vi "ATM main.vi"() -> ()   [LabVIEW 2017]
doc: "This VI is the main VI of the ATM simulator. This VI performs the all operation of the ATM machine as per the requirements."
panel:
  out "String":string
  out "Error Out":errorcluster
  in  "Mehr Buttons":cluster{"L1":bool, "L2":bool, "L3":bool}
  out "Display":string
  out "Menü 2":T1
  out "Menü 1":T1
  in  "Buttons":cluster{"L1":bool, "L2":bool, "L3":bool}
  in  "Enter":bool
  in  "Eingabe  Feld":string
  in  "Karteneingabe":bool
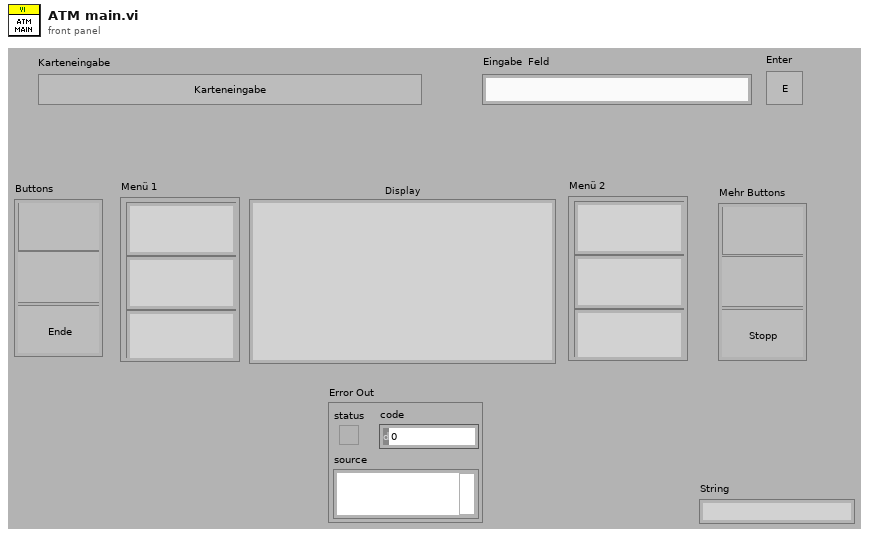
[diagram p1: front panel]
types:
  T1 = cluster{"LM1":string, "LM2":string, "LM3":string}
  T2 = enum8{"Enabled", "Disabled", "Disabled and Grayed Out"}
  T3 = cluster{"amount":string[], "accno":string[], "lst name":string[], "first name":string[]}
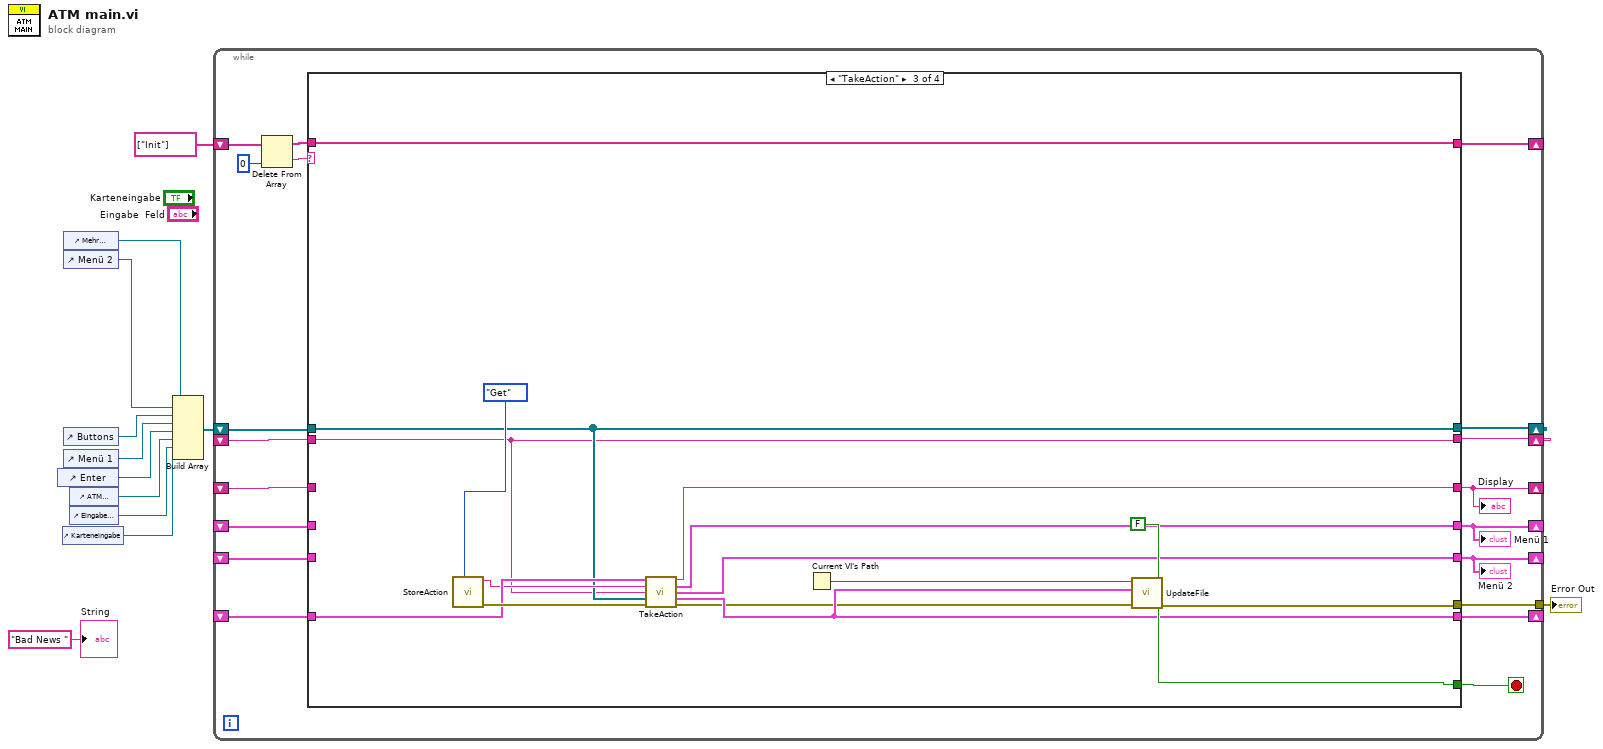
[diagram p0: block diagram]
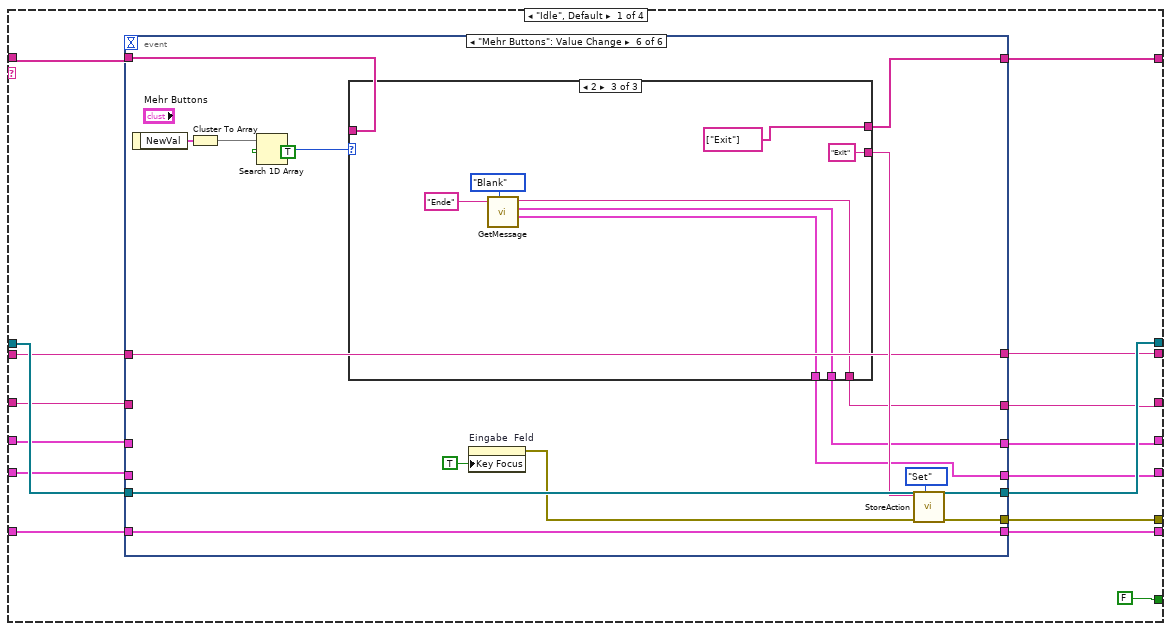
[diagram p2: hidden frame]
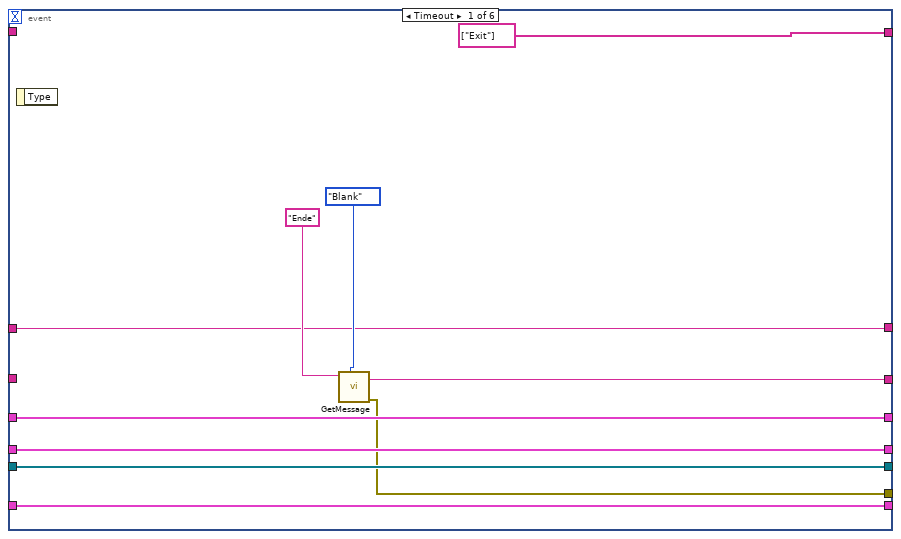
[diagram p3: hidden frame]
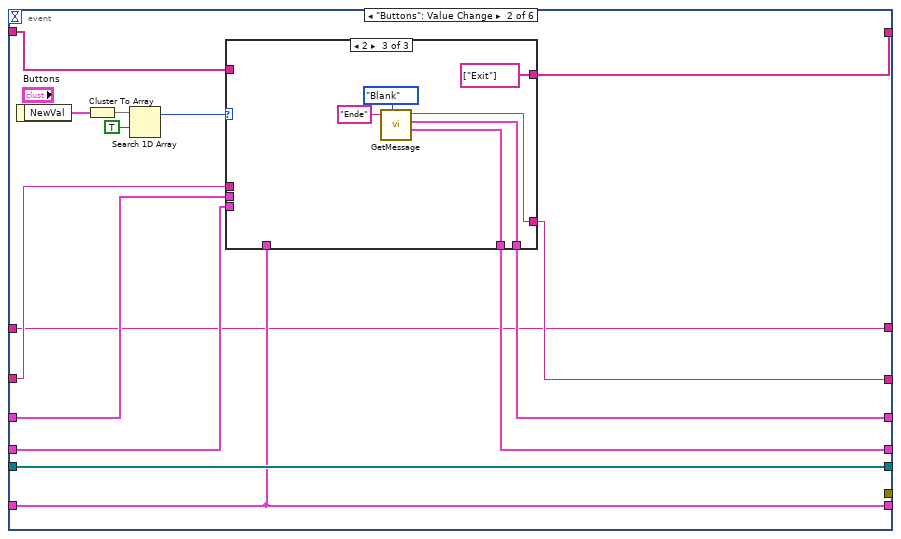
[diagram p4: hidden frame]
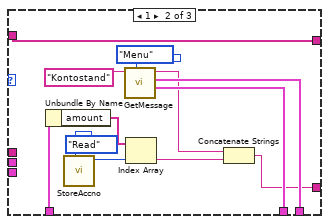
[diagram p6: hidden frame]
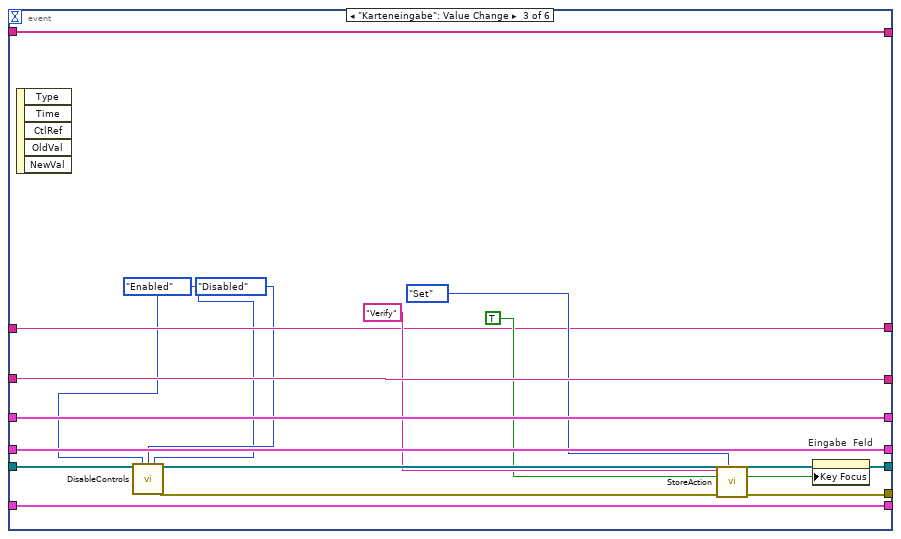
[diagram p7: hidden frame]
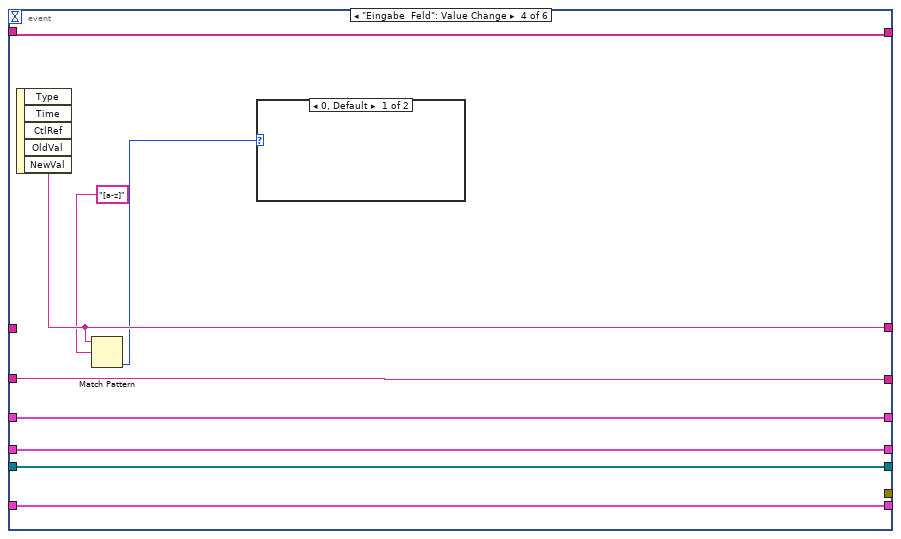
[diagram p8: hidden frame]
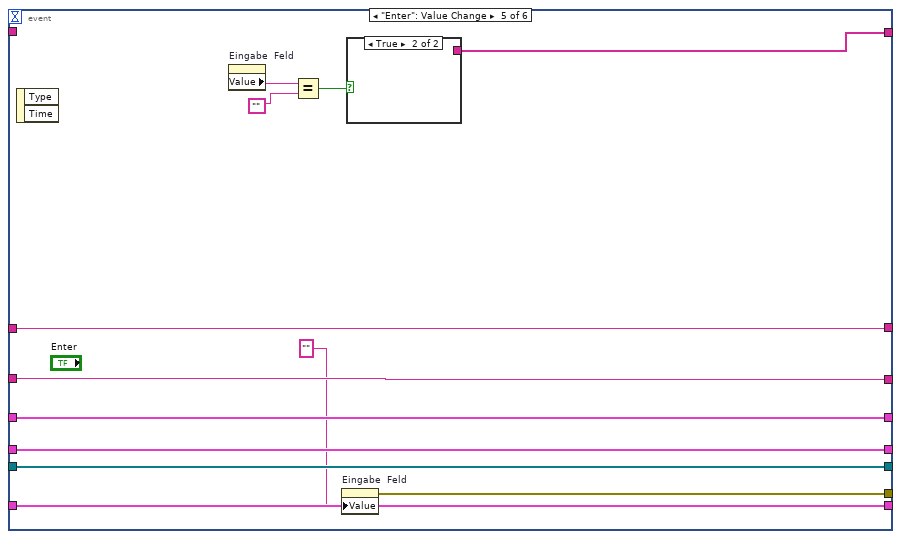
[diagram p10: hidden frame]
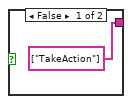
[diagram p11: hidden frame]
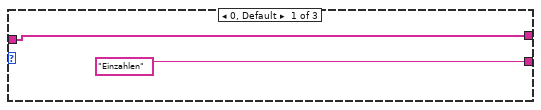
[diagram p12: hidden frame]
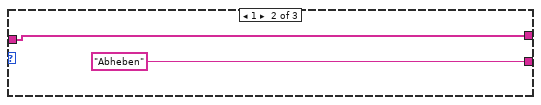
[diagram p13: hidden frame]
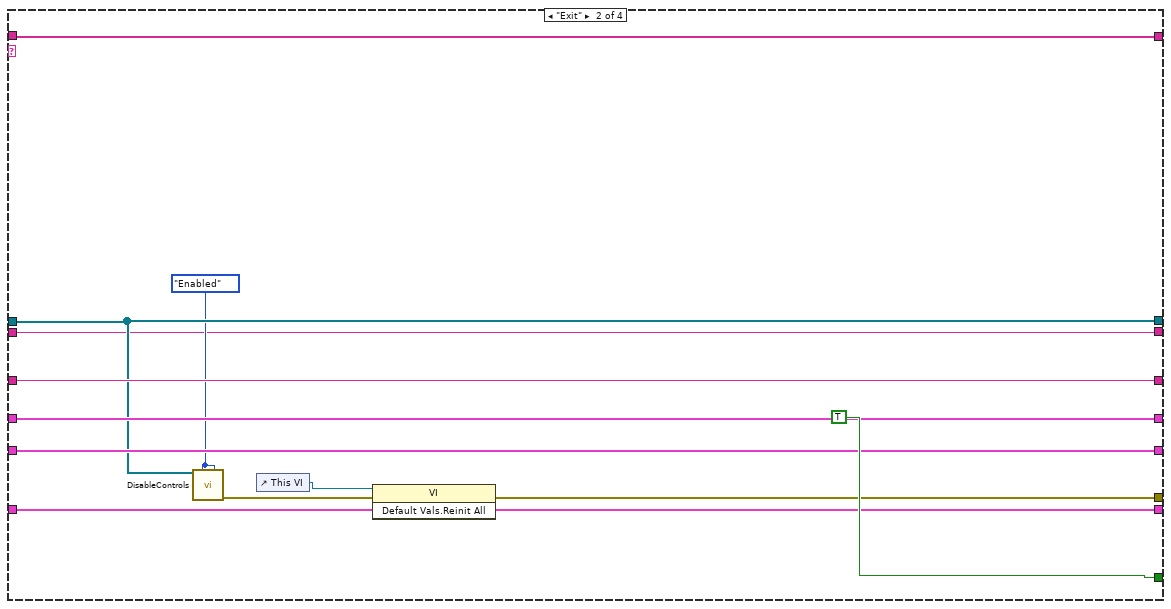
[diagram p14: hidden frame]
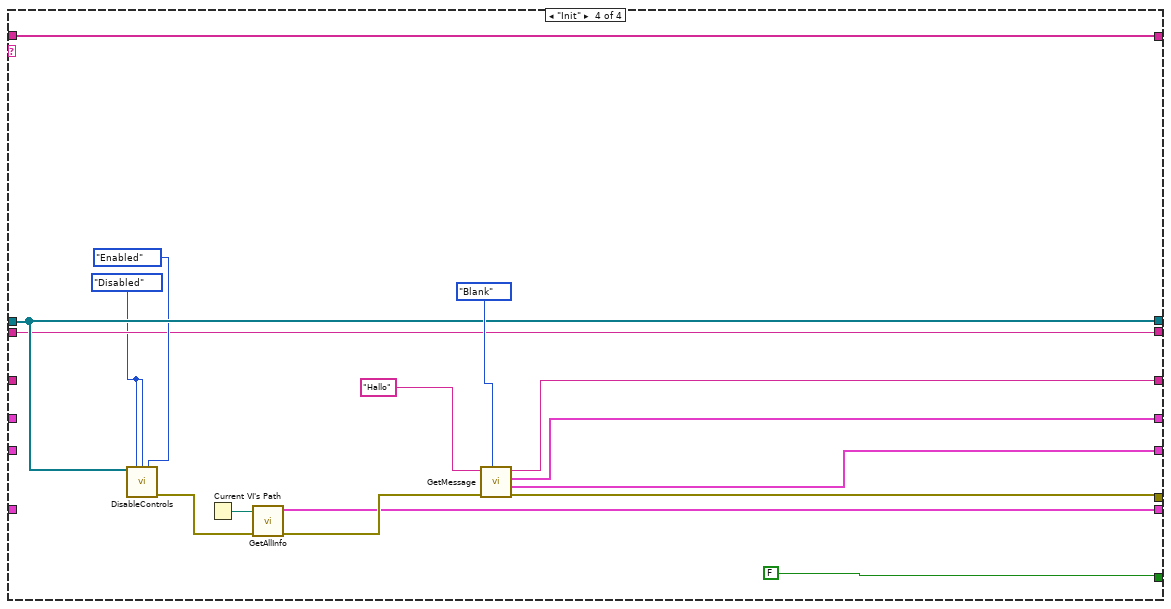
[diagram p15: hidden frame]
diagram:
  n1 = control-ref of="Enter"() -> (w7:refnum<vi>)
  n2 = control-ref of="Karteneingabe"() -> (w2:refnum<vi>)
  n3 = control-ref of="Mehr Buttons"() -> (w11:refnum<vi>)
  n4 = control-ref of="Menü 2"() -> (w10:refnum<vi>)
  n5 = control-ref of="Buttons"() -> (w9:refnum<vi>)
  n6 = control-ref of="Menü 1"() -> (w8:refnum<vi>)
  n7 = control-ref of="ATM Messages"() -> (w6:refnum<vi>)
  n8 = control-ref of="Eingabe  Feld"() -> (w5:refnum<vi>)
  n9 = Build Array(w11, w10, w9, w8, w7, w6, w5, w2) -> (w4:refnum<vi>[])
  n10 = while {
    shift-right: [w24] -> _
    shift-left: string[] ["Init"] -> [w31]
    shift-right: [w26] -> _
    shift-left: w4 -> [w27]
    shift-right: [w20] -> _
    shift-left: _ -> [w19]
    shift-right: [w21] -> _
    shift-left: _ -> [w18]
    shift-right: [w22] -> _
    shift-left: _ -> [w17]
    shift-right: [w16] -> _
    shift-left: _ -> [w15]
    shift-right: [w14] -> _
    shift-left: _ -> [w13]
    tunnel: [w23] -> w3
    stop <- w28 stop-if-true
    n11 = Delete From Array(array=w31, index=0) -> (deleted portion=w29:string, array with subset deleted=w25:string[])  [unwired: 1 in]
    n12 = case shown="\"TakeAction\"" w29 {
      tunnel: [FALSE TRUE FALSE FALSE] -> w28
      tunnel: w27 -> [w47 w164 w172 w190]
      tunnel: [w46 w164 w172 w190] -> w26
      tunnel: w25 -> [w34 w169 w184 w200]
      tunnel: [w35 w169 w184 w200] -> w24
      tunnel: [w44 w160 w177 w196] -> w23
      tunnel: [w42 w168 w181 w195] -> w20
      tunnel: [w40 w167 w180 w194] -> w21
      tunnel: [w38 w166 w179 w193] -> w22
      tunnel: w19 -> [w43 w168 _ _]
      tunnel: w18 -> [w41 w167 _ _]
      tunnel: w17 -> [w39 w166 _ _]
      tunnel: [w36 w165 w175 w188] -> w16
      tunnel: w15 -> [w37 w165 w178 _]
      tunnel: [w33 w159 w171 w187] -> w14
      tunnel: w13 -> [w32 w159 w171 w187]
      frame "Idle", Default {
        n13 = event shown="[5] \"Mehr Buttons\": Value Change" {
          selector: _ -> [_ _ _ _ _ _]
          dyn-events: _ -> [_ _ _ _ _ _]
          timeout: _ -> [_ _ _ _ _ _]
          tunnel: w47 -> [w57 w72 w105 w117 w129 w147]
          tunnel: [w57 w72 w105 w117 w129 w147] -> w46
          tunnel: [w48 _ w102 _ w123 w134] -> w44
          tunnel: w43 -> [_ w63 w108 w116 w128 _]
          tunnel: [w51 w66 w108 w116 w128 w133] -> w42
          tunnel: w41 -> [w56 w62 w107 w115 w127 _]
          tunnel: [w56 w65 w107 w115 w127 w132] -> w40
          tunnel: w39 -> [w55 w61 w106 w114 w126 _]
          tunnel: [w55 w64 w106 w114 w126 w131] -> w38
          tunnel: w37 -> [w54 w67 w104 w113 w125 w146]
          tunnel: [w54 w67 w104 w113 w125 w146] -> w36
          tunnel: [string[] ["Exit"] w60 w99 w112 w118 w138] -> w35
          tunnel: w34 -> [_ w59 w99 w112 _ w137]
          tunnel: [w49 w58 w97 w111 w122 w136] -> w33
          tunnel: w32 -> [w49 w58 w97 _ w122 w136]
          event Timeout {
            n14 = event-data() -> ()  [unwired: 1 in, 1 out]
            n15 = call "GetMessage.vi"("Action"=enum16{"Blank", "Menu"}."Blank", "Message Type"="Ende") -> ("Error Out"=w48:errorcluster, "Get Message"=w51:string)  [unwired: 6 in, 2 out]
          }
          event "Buttons": Value Change {
            n16 = event-data() -> ("NewVal"=w71:cluster{"L1":bool, "L2":bool, "L3":bool})  [unwired: 1 in]
            n17 = Cluster To Array(cluster=w71) -> (array=w70:bool[])
            n18 = Search 1D Array(1D array=w70, element=TRUE) -> (index of element=w68:i32)  [unwired: 1 in]
            n19 = case shown="2" w68 {
              tunnel: w67 -> [_ w86 _]
              tunnel: [w76 w79 w92] -> w66
              tunnel: [w75 w81 w91] -> w65
              tunnel: [w74 w80 w90] -> w64
              tunnel: w63 -> [w76 _ _]
              tunnel: w62 -> [w75 _ _]
              tunnel: w61 -> [w74 _ _]
              tunnel: [w73 w78 string[] ["Exit"]] -> w60
              tunnel: w59 -> [w73 w78 _]
              frame 0, Default {
              }
              frame 1 {
                n20 = Unbundle By Name(w86) -> ("amount"=w83:string[])
                n21 = call "StoreAccno.vi"("Enum"=enum16{"Read", "Write"}."Read") -> ("Read"=w84:i32)  [unwired: 10 in]
                n22 = call "GetMessage.vi"("Action"=enum16{"Blank", "Menu"}."Menu", "Message Type"="Kontostand") -> ("Right Menu"=w80:cluster{"R1":string, "R2":string, "R3":string}, "Left menu"=w81:cluster{"L1":string, "L2":string, "L3":string}, "Get Message"=w77:string)  [unwired: 6 in, 1 out]
                n23 = Index Array(array=w83, index=w84) -> (element=w82:string)
                n24 = Concatenate Strings(w77, w82) -> (w79:string)
              }
              frame 2 {
                n25 = call "GetMessage.vi"("Action"=enum16{"Blank", "Menu"}."Blank", "Message Type"="Ende") -> ("Right Menu"=w90:cluster{"R1":string, "R2":string, "R3":string}, "Left menu"=w91:cluster{"L1":string, "L2":string, "L3":string}, "Get Message"=w92:string)  [unwired: 6 in, 1 out]
              }
            }
          }
          event "Karteneingabe": Value Change {
            w95 = T2."Enabled" ("Disabled")
            n26 = event-data() -> ()  [unwired: 1 in, 5 out]
            n27 = call "DisableControls.vi"("Array"=w105, "User Input"=w95, "Menu action"=T2."Disabled" ("Disabled"), "Card Simulator"=w95) -> ("Error Out"=w103:errorcluster)  [unwired: 11 in]
            n28 = call "StoreAction.vi"("Enum"=enum16{"Set", "Get"}."Set", "Error in"=w103, "Write action"="Verify") -> ("Error out"=w102:errorcluster)  [unwired: 7 in, 1 out]
            n29 = property on="Eingabe  Feld" class="Str"("Key Focus"=TRUE) -> ()  [unwired: 2 in, 2 out]
          }
          event "Eingabe  Feld": Value Change {
            n30 = event-data() -> ("NewVal"=w111:string)  [unwired: 1 in, 4 out]
            n31 = Match Pattern(string=w111, regular expression="[a-z]") -> (offset past match=w109:i32)  [unwired: 1 in, 3 out]
            n32 = case shown="0, Default" w109 {
              frame 0, Default {
              }
              frame -1 {
              }
            }
          }
          event "Enter": Value Change {
            n33 = event-data() -> ()  [unwired: 1 in, 2 out]
            n34 = property on="Eingabe  Feld" class="Str"() -> ("Value"=w121:string)  [unwired: 2 in, 2 out]
            n35 = Equal?(x=w121, y="") -> (x = y?=w119:bool)
            n36 = property on="Eingabe  Feld" class="Str"("Value"="" ("User Input")) -> (error out=w123:errorcluster)  [unwired: 2 in, 1 out]
            n37 = case shown="True" w119 {
              tunnel: [string[] ["TakeAction"] _] -> w118
              frame False {
              }
              frame True {
              }
            }
          }
          event "Mehr Buttons": Value Change {
            n38 = event-data() -> ("NewVal"=w145:cluster{"L1":bool, "L2":bool, "L3":bool})  [unwired: 1 in]
            n39 = Cluster To Array(cluster=w145) -> (array=w144:bool[])
            n40 = Search 1D Array(1D array=w144, element=TRUE) -> (index of element=w142:i32)  [unwired: 1 in]
            n41 = case shown="2" w142 {
              tunnel: ["Einzahlen" "Abheben" "Exit"] -> w140
              tunnel: [w148 w150 string[] ["Exit"]] -> w138
              tunnel: w137 -> [w148 w150 _]
              tunnel: [_ _ w156] -> w133
              tunnel: [_ _ w155] -> w132
              tunnel: [_ _ w154] -> w131
              frame 0, Default {
              }
              frame 1 {
              }
              frame 2 {
                n42 = call "GetMessage.vi"("Action"=enum16{"Blank", "Menu"}."Blank", "Message Type"="Ende") -> ("Right Menu"=w154:cluster{"R1":string, "R2":string, "R3":string}, "Left menu"=w155:cluster{"L1":string, "L2":string, "L3":string}, "Get Message"=w156:string)  [unwired: 6 in, 1 out]
              }
            }
            n43 = property on="Eingabe  Feld" class="Str"("Key Focus"=TRUE) -> (error out=w135:errorcluster)  [unwired: 2 in, 1 out]
            n44 = call "StoreAction.vi"("Enum"=enum16{"Set", "Get"}."Set", "Error in"=w135, "Write action"=w140) -> ("Error out"=w134:errorcluster)  [unwired: 7 in, 1 out]
          }
        }
      }
      frame "Exit" {
        w163 = T2."Enabled" ("User Input")
        n45 = call "DisableControls.vi"("Array"=w164, "User Input"=w163, "Card Simulator"=w163) -> ("Error Out"=w161:errorcluster)  [unwired: 12 in]
        n46 = control-ref of="This VI"() -> (w162:refnum<vi>)
        n47 = invoke class="VI" method="Default Vals.Reinit All"(reference=w162, error in=w161) -> (error out=w160:errorcluster)  [unwired: 1 in, 2 out]
      }
      frame "TakeAction" {
        n48 = call "StoreAction.vi"("Enum"=enum16{"Set", "Get"}."Get") -> ("Error out"=w182:errorcluster, "Read action"=w174:string)  [unwired: 9 in]
        n49 = call "TakeAction.vi"("Account Info"=w178, "Action"=w174, "User input"=w171, "Array"=w172, "Error in"=w182) -> ("Get Message"=w181:string, "Left menu"=w180:cluster{"L1":string, "L2":string, "L3":string}, "Right Menu"=w179:cluster{"R1":string, "R2":string, "R3":string}, "Updated acc info"=w175:T3, "Error out"=w173:errorcluster)  [unwired: 6 in]
        n50 = Current VI's Path() -> (path=w176:path)
        n51 = call "UpdateFile.vi"("error in (no error)"=w173, "Account Info"=w175, "path"=w176) -> ("error out"=w177:errorcluster)  [unwired: 8 in]
      }
      frame "Init" {
        w186 = T2."Disabled" ("Action user Menu")
        n52 = call "DisableControls.vi"("Array"=w190, "User Input"=w186, "Menu action"=w186, "Card Simulator"=T2."Enabled" ("Action user Menu")) -> ("Error Out"=w199:errorcluster)  [unwired: 11 in]
        n53 = Current VI's Path() -> (path=w198:path)
        n54 = call "GetAllInfo.vi"("Error in"=w199, "base path"=w198) -> ("Error out"=w197:errorcluster, "Account Info"=w188:T3)  [unwired: 8 in]
        n55 = call "GetMessage.vi"("Action"=enum16{"Blank", "Menu"}."Blank", "Error in"=w197, "Message Type"="Hallo") -> ("Error Out"=w196:errorcluster, "Right Menu"=w193:cluster{"R1":string, "R2":string, "R3":string}, "Left menu"=w194:cluster{"L1":string, "L2":string, "L3":string}, "Get Message"=w195:string)  [unwired: 5 in]
      }
    }
    "Display" <- w20
    "Menü 1" <- w21
    "Menü 2" <- w22
  }
  "Error Out" <- w3
  "String" <- "Bad News " ("String")
